vi "总磷总氮质控参数设置.vi"(11 "质控参数设置":T1) -> (2 "质控参数设置 2":T1, 3 "check？":bool)   [LabVIEW 2016, in "斯坦道氨氮.lvlib"]
uses:
  <vilib>/Utility/miscctls.llb/LVPointTypeDef.ctl
panel:
  in  "质控参数":i32(listbox)
  in  "取消":bool
  in  "确定":bool
  # "质控参数设置"
  # "质控参数设置"
  # "总氮"
  # "COD"
  # "氨氮"
  # "监测参数"
  # "总磷"
  # "跨度值"
  # "零点核查标准液浓度"
  # "跨度核查标准液浓度"
  # "标样核查标准液浓度"
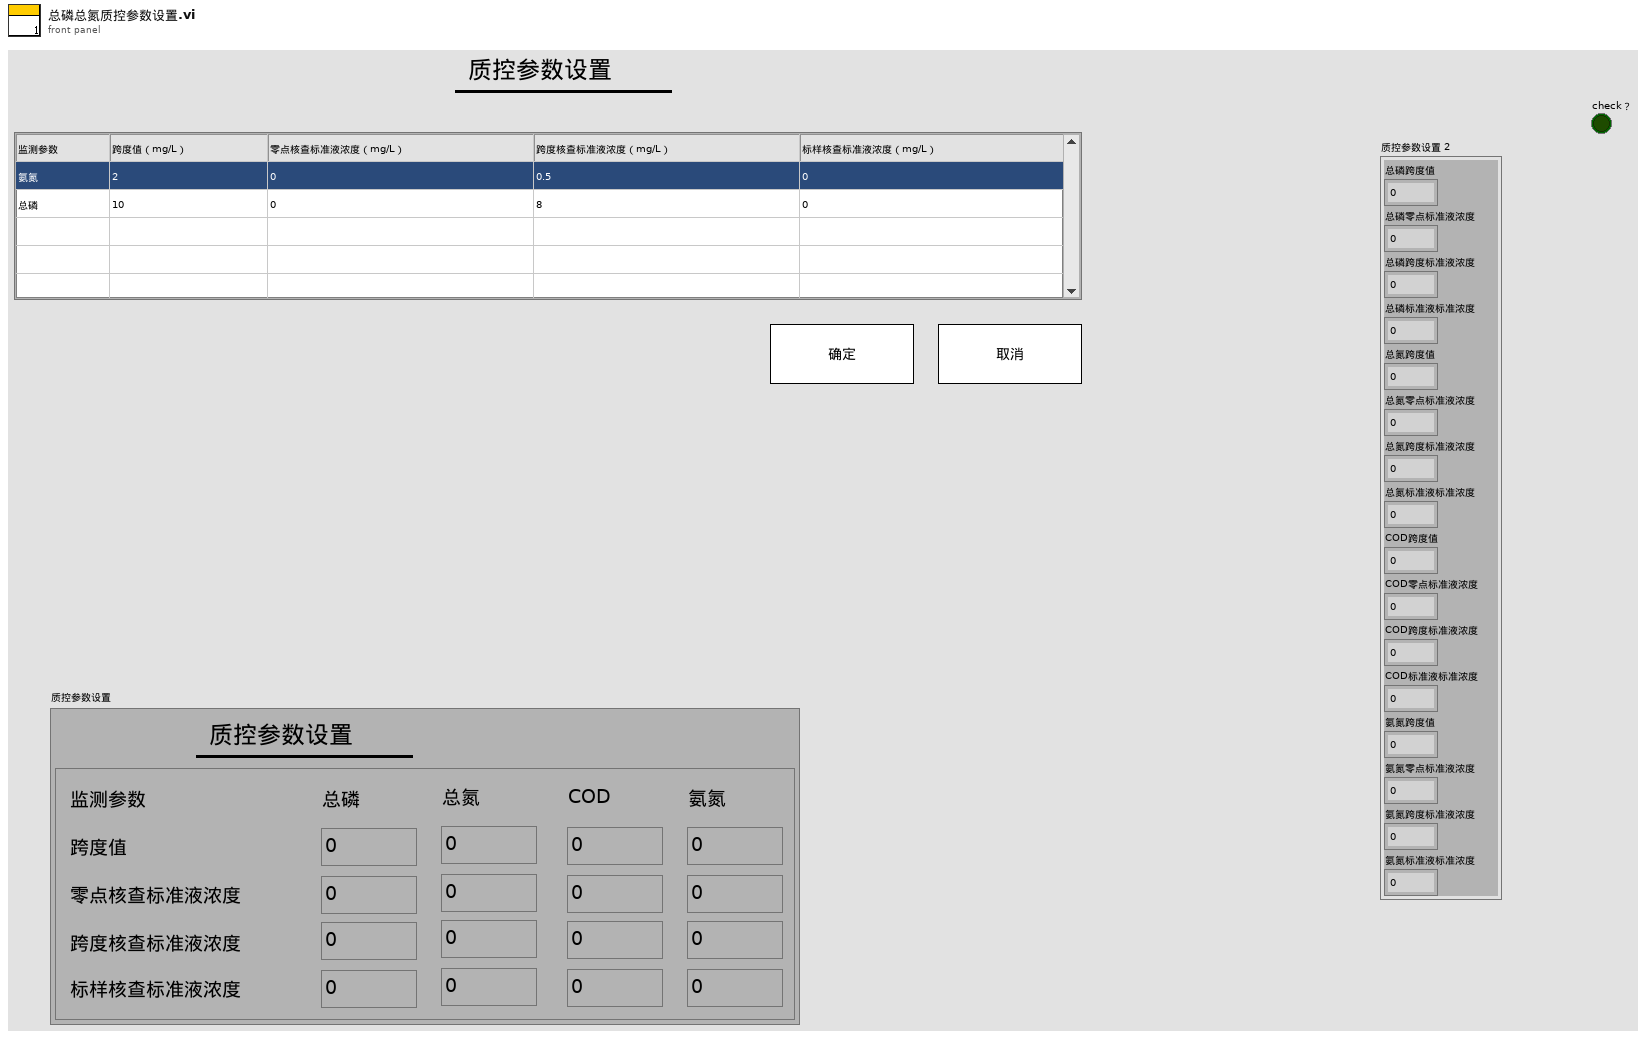
[diagram p1: front panel]
types:
  T1 = cluster{"总磷跨度值":dbl, "总磷零点标准液浓度":dbl, "总磷跨度标准液浓度":dbl, "总磷标准液标准浓度":dbl, "总氮跨度值":dbl, "总氮零点标准液浓度":dbl, "总氮跨度标准液浓度":dbl, "总氮标准液标准浓度":dbl, "COD跨度值":dbl, "COD零点标准液浓度":dbl, "COD跨度标准液浓度":dbl, "COD标准液标准浓度":dbl, "氨氮跨度值":dbl, "氨氮零点标准液浓度":dbl, "氨氮跨度标准液浓度":dbl, "氨氮标准液标准浓度":dbl}
  T2 = typedef "LVPointTypeDef.ctl" = cluster{"Horizontal":i16, "Vertical":i16}
  T3 = cluster{"COD":bool, "氨氮":bool, "总氮":bool, "总磷":bool}
  T4 = typedef "LVPoint32TypeDef.ctl" = cluster{"Horizontal":i32, "Vertical":i32}
  T5 = typedef "LVRowAndColumnTypeDef.ctl" = cluster{"Row":i32, "Column":i32}
  T6 = cluster{"质控参数设置[0]":dbl, "质控参数设置[1]":dbl, "质控参数设置[2]":dbl, "质控参数设置[3]":dbl, "质控参数设置[4]":dbl, "质控参数设置[5]":dbl, "质控参数设置[6]":dbl, "质控参数设置[7]":dbl, "质控参数设置[8]":dbl, "质控参数设置[9]":dbl, "质控参数设置[10]":dbl, "质控参数设置[11]":dbl, "质控参数设置[12]":dbl, "质控参数设置[13]":dbl, "质控参数设置[14]":dbl, "质控参数设置[15]":dbl}
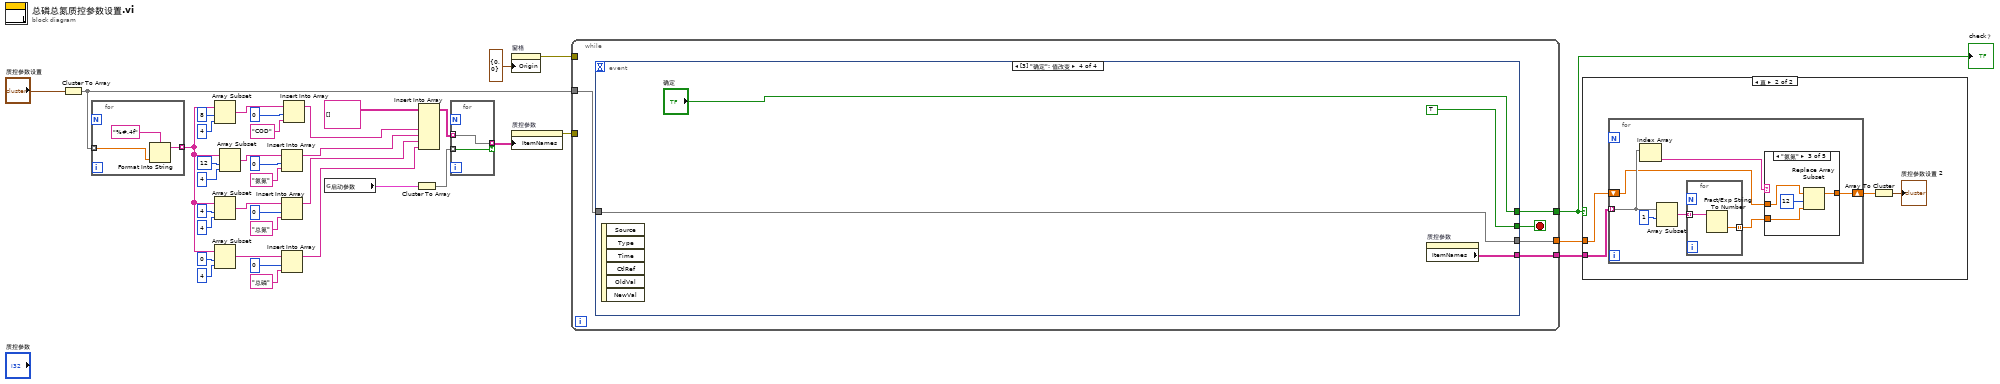
[diagram p0: block diagram]
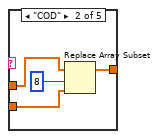
[diagram p4: hidden frame]
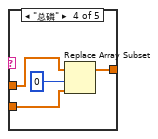
[diagram p5: hidden frame]
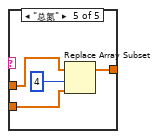
[diagram p6: hidden frame]
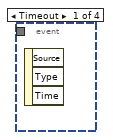
[diagram p7: hidden frame]
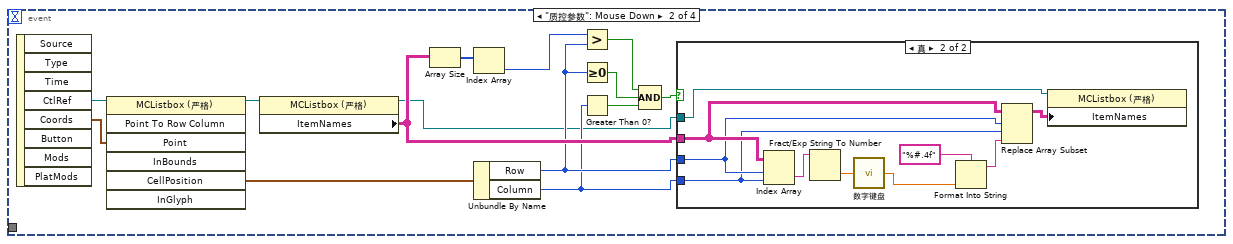
[diagram p8: hidden frame]
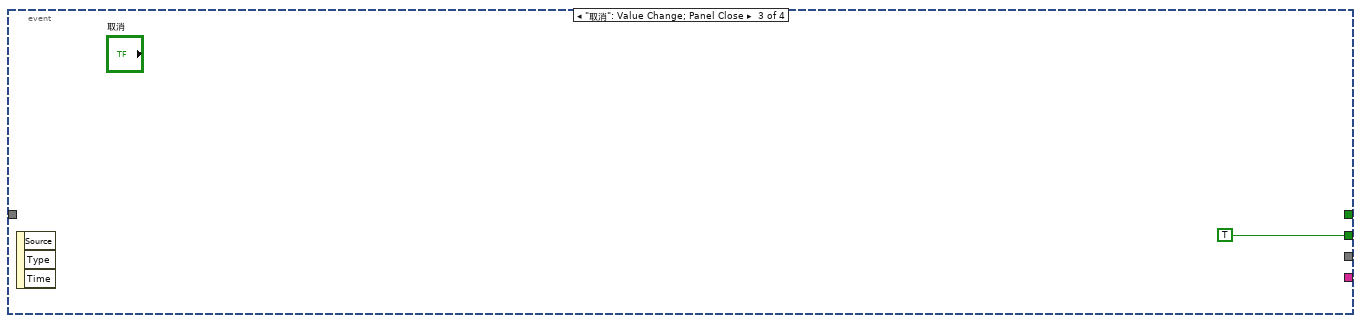
[diagram p10: hidden frame]
diagram:
  n1 = Cluster To Array(cluster="质控参数设置") -> (array=w4:dbl[])
  n2 = for {
    tunnel: w4 -> [w40] mode=indexing
    tunnel: [w39] -> w15 mode=indexing
    n3 = Format Into String(format string="%#.4f" ("格式字符串"), w40) -> (resulting string=w39:string)  [unwired: 2 in, 1 out]
  }
  n4 = Array Subset(array=w15, index=8 ("索引"), length=4 ("长度")) -> (w23:string[])
  n5 = Array Subset(array=w15, index=4 ("索引"), length=4 ("长度")) -> (w28:string[])
  n6 = Array Subset(array=w15, index=0 ("索引"), length=4 ("长度")) -> (w33:string[])
  n7 = Array Subset(array=w15, index=12 ("索引"), length=4 ("长度")) -> (w18:string[])
  n8 = Insert Into Array(array=w18, index=0 ("索引"), new element="氨氮" ("新元素/子数组")) -> (w12:string[])
  n9 = Insert Into Array(array=w28, index=0 ("索引"), new element="总氮" ("新元素/子数组")) -> (w11:string[])
  n10 = Insert Into Array(array=w33, index=0 ("索引"), new element="总磷" ("新元素/子数组")) -> (w10:string[])
  n11 = Insert Into Array(array=w23, index=0 ("索引"), new element="COD" ("新元素/子数组")) -> (w13:string[])
  n12 = global read "总磷总氮断电保存全局变量.vi" "启动参数"() -> (w7:T3)
  n13 = Cluster To Array(cluster=w7) -> (array=w6:bool[])
  n14 = Insert Into Array(array=string[][] [], new element #1=w13, new element #2=w12, new element #3=w11, new element #4=w10) -> (w8:string[][])  [unwired: 2 in]
  n15 = for {
    tunnel: w8 -> [w43] mode=indexing
    tunnel: w6 -> [w42] mode=indexing
    tunnel: [w43] -> w5 mode=indexing if=w42
  }
  n16 = property on="窗格" class="Pane"("Origin"=T2 {"Horizontal"=0, "Vertical"=0} ("原点")) -> (error out=w37:errorcluster)  [unwired: 2 in, 1 out]
  n17 = property on="质控参数" class="MCListbox (严格)"("ItemNames"=w5) -> (error out=w9:errorcluster)  [unwired: 2 in, 1 out]
  n18 = while {
    tunnel: w37 -> [_]
    tunnel: [w47] -> w1
    tunnel: w9 -> [_]
    tunnel: w4 -> [w46]
    tunnel: [w45] -> w3
    tunnel: [w44] -> w2
    stop <- w48 stop-if-true
    n19 = event shown="[3] \"确定\": 值改变" {
      selector: _ -> [_ _ _ _]
      dyn-events: _ -> [_ _ _ _]
      timeout: _ -> [_ _ _ _]
      tunnel: [_ _ TRUE TRUE] -> w48
      tunnel: [_ _ _ "确定"] -> w47
      tunnel: w46 -> [_ _ _ w75]
      tunnel: [_ _ _ w75] -> w45
      tunnel: [_ _ _ w74] -> w44
      event Timeout {
        n20 = event-data() -> ()  [unwired: 1 in, 3 out]
      }
      event "质控参数": Mouse Down {
        n21 = event-data() -> ("CtlRef"=w62:refnum<vi>, "Coords"=w61:T4)  [unwired: 1 in, 6 out]
        n22 = invoke class="MCListbox (严格)" method="Point To Row Column"(reference=w62, "Point"=w61) -> (reference out=w60:refnum<vi>, "CellPosition"=w59:T5)  [unwired: 5 in, 5 out]
        n23 = property class="MCListbox (严格)"(reference=w60) -> (reference out=w49:refnum<vi>, "ItemNames"=w52:string[][])  [unwired: 1 in, 1 out]
        n24 = Array Size(array=w52) -> (size(s)=w56:i32[])
        n25 = Index Array(array=w56) -> (element=w55:i32)  [unwired: 1 in]
        n26 = Unbundle By Name(w59) -> ("Row"=w51:i32, "Column"=w50:i32)
        n27 = Greater?(x=w55, y=w51) -> (0:w54:bool)
        n28 = Greater Or Equal To 0?(x=w51) -> (x >= 0?=w53:bool)
        n29 = Greater Than 0?(x=w50) -> (x > 0?=w58:bool)
        n30 = Compound Arithmetic op=AND ("复合运算")(w54, w53, w58) -> (w57:bool)
        n31 = case shown="真" w57 {
          tunnel: w52 -> [_ w68]
          tunnel: w51 -> [_ w67]
          tunnel: w50 -> [_ w66]
          tunnel: w49 -> [_ w63]
          frame False {
          }
          frame True {
            n32 = Index Array(array=w68, index (row)=w67, index (col)=w66) -> (element=w72:string)
            n33 = Fract/Exp String To Number(string=w72) -> (number=w71:dbl)  [unwired: 3 in, 1 out]
            n34 = call "数字键盘.vi"("OldNumber"=w71) -> ("NewNumber"=w70:dbl)
            n35 = Format Into String(format string="%#.4f" ("格式字符串"), w70) -> (resulting string=w65:string)  [unwired: 2 in, 1 out]
            n36 = Replace Array Subset(array=w68, new element=w65, index (row)=w67, index (col)=w66) -> (w64:string[][])
            n37 = property class="MCListbox (严格)"(reference=w63, "ItemNames"=w64) -> ()  [unwired: 1 in, 2 out]
          }
        }
      }
      event "取消": Value Change; Panel Close {
        n38 = event-data() -> ()  [unwired: 1 in, 3 out]
      }
      event "确定": Value Change {
        n39 = event-data() -> ()  [unwired: 1 in, 6 out]
        n40 = property on="质控参数" class="MCListbox (严格)"() -> ("ItemNames"=w74:string[][])  [unwired: 2 in, 2 out]
      }
    }
  }
  "check？" <- w1
  n41 = case shown="真" w1 {
    tunnel: w3 -> [_ w81]
    tunnel: w2 -> [_ w80]
    frame False {
    }
    frame True {
      n42 = for {
        tunnel: w80 -> [w87] mode=indexing
        shift-right: [w82] -> w79
        shift-left: w81 -> [w83]
        n43 = Index Array(array=w87) -> (element=w88:string)  [unwired: 1 in]
        n44 = Array Subset(array=w87, index=1 ("索引")) -> (w85:string[])  [unwired: 1 in]
        n45 = for {
          tunnel: w85 -> [w90] mode=indexing
          tunnel: [w89] -> w84 mode=indexing
          n46 = Fract/Exp String To Number(string=w90) -> (number=w89:dbl)  [unwired: 3 in, 1 out]
        }
        n47 = case shown="\"氨氮\"" w88 {
          tunnel: w84 -> [_ w94 w98 w102 w106]
          tunnel: w83 -> [w91 w95 w99 w103 w107]
          tunnel: [w91 w93 w97 w101 w105] -> w82
          frame Default {
          }
          frame "COD" {
            n48 = Replace Array Subset(array=w95, new element=w94, index=8 ("索引")) -> (w93:dbl[])
          }
          frame "氨氮" {
            n49 = Replace Array Subset(array=w99, new element=w98, index=12 ("索引")) -> (w97:dbl[])
          }
          frame "总磷" {
            n50 = Replace Array Subset(array=w103, new element=w102, index=0 ("索引")) -> (w101:dbl[])
          }
          frame "总氮" {
            n51 = Replace Array Subset(array=w107, new element=w106, index=4 ("索引")) -> (w105:dbl[])
          }
        }
      }
      n52 = Array To Cluster(array=w79) -> (cluster=→"质控参数设置 2":T6)
    }
  }
